vi "worksheet insert button.vi"(7 "options":T1, 8 "error in (no error)":errorcluster, 9 "col":u16, 10 "row":u32, 11 "worksheet":u32) -> (0 "error out":errorcluster, 3 "function return":u32(ring), 5 "options out":T1)   [LabVIEW 8.6]
doc: "lxw_error worksheet_insert_button(lxw_worksheet worksheet, lxw_row_t row, lxw_col_t col, lxw_button_options *options);"
uses:
  pending_lvxlsxwriter/xlsxwriter.dll
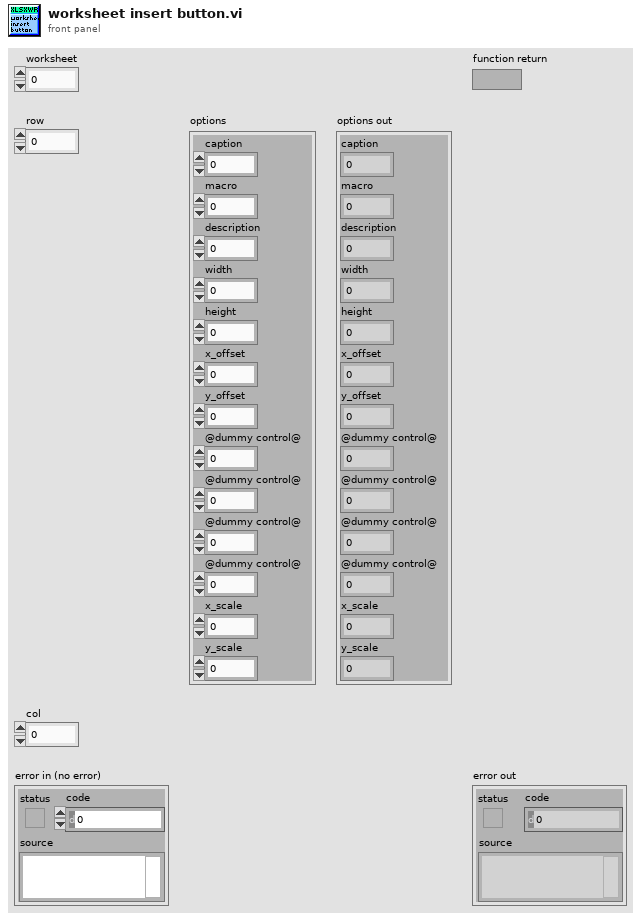
[diagram p1: front panel]
types:
  T1 = cluster{"caption":u32, "macro":u32, "description":u32, "width":u32, "height":u32, "x_offset":i32, "y_offset":i32, "@dummy control@":i8, "@dummy control@":i8, "@dummy control@":i8, "@dummy control@":i8, "x_scale":dbl, "y_scale":dbl}
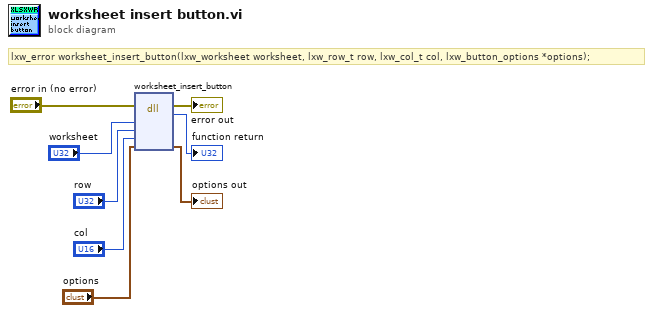
[diagram p0: block diagram]
diagram:
  # "lxw_error worksheet_insert_button(lxw_worksheet worksheet, lxw_row_t row, lxw_col_t col, lxw_button_options *options);"
  n1 = dll-call lib="C:/Users/WDAGUtilityAccount/Desktop/pending_lvxlsxwriter/xlsxwriter.*" fn="worksheet_insert_button"(error in="error in (no error)", "worksheet"="worksheet", "row"="row", "col"="col", "options"="options") -> (error out=→"error out":errorcluster, →"function return":u32, "options"=→"options out":T1)  [unwired: 5 in, 1 out]
